vi "Read_StoreImage.vi"() -> (3 "STORE_IMAGE":bool)   [LabVIEW 2023, in "Cam Data.lvlib"]
uses:
  Cam Data.lvlib
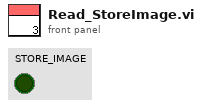
[diagram p1: front panel]
types:
  T1 = cluster{"Address IP":string, "Rack":i32, "Slot ":i32, "DB Number":i32, "Start":i32, "Amount":i32}
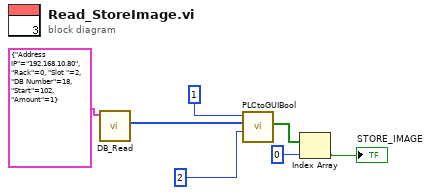
[diagram p0: block diagram]
diagram:
  n1 = call "DB_Read.vi"("Input Params"=T1 {"Address IP"="192.168.10.80", "Rack"=0, "Slot "=2, "DB Number"=18, "Start"=102, "Amount"=1}) -> ("Data"=w3:u8[])  [unwired: 8 in, 2 out]
  n2 = call "PLCtoGUIBool.vi"("SubOffset"=u16 2, "DB Input Vals"=w3, "DB Val Qty"=u16 1) -> ("BoolValue"=w5:bool[])  [unwired: 8 in]
  n3 = Index Array(array=w5, index=0) -> (element=→"STORE_IMAGE":bool)
